vi "GetCameraData.vi"(7 "LabVIEW Web Service Request":refnum<class "Web Request.lvclass">) -> ()   [LabVIEW 2017]
uses:
  <vilib>/wsapi/Web Request.lvclass
  DataAccessors/action.ctl
  DataAccessors/cameraData.ctl
  DataAccessors/VisionWebServiceData.lvlib
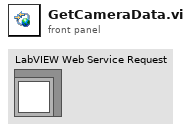
[diagram p1: front panel]
types:
  T1 = typedef "VisionWebServiceData.lvlib/action.ctl" = enum16{"Get", "Set"}
  T2 = typedef "VisionWebServiceData.lvlib/cameraData.ctl" = cluster{"Width":i32, "Height":i32, "Data":string}
  T3 = typedef "IrAcquisition.lvlib/camera.ctl" = cluster{"Name":string, "ChannelId":string, "CameraId":string, "SerialNumber":string, "Unit":string, "IMAQSession":T4, "InterfaceName":string, "RawImage":T5, "ScaledImage":T5, "TestPanelImage":T5, "Map":T6, "InDeviceModel":bool}
  T4 = typedef "IMAQdx.ctl" = refnum<k21>
  T5 = typedef "IMAQ Image.ctl" = refnum<image>
  T6 = typedef "PointValueMap.lvlib/PointMap.ctl" = refnum<data-value>
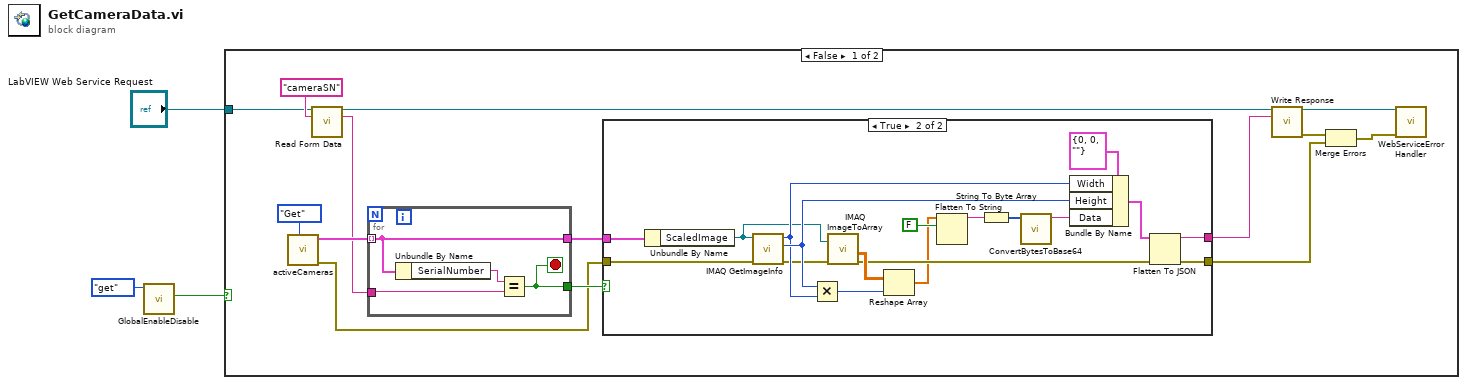
[diagram p0: block diagram]
diagram:
  n1 = call "GlobalEnableDisable.vi"("action"=enum16{"init", "set", "get"}."get") -> ("DisableDeviceWebService"=w1:bool)  [unwired: 10 in]
  n2 = case shown="False" w1 {
    tunnel: "LabVIEW Web Service Request" -> [w16 _]
    frame False {
      n3 = call "activeCameras.vi"("action"=action."Get") -> ("error out"=w7:errorcluster, "cameras"=w14:T3[])  [unwired: 9 in]
      n4 = call <vilib>:"Read Form Data.vi"("LabVIEW Web Service Request"=w16, "key"="cameraSN") -> ("LabVIEW Web Service Request out"=w13:refnum<class "Web Request.lvclass">, "value"=w8:string)  [unwired: 10 in, 2 out]
      n5 = for {
        tunnel: w14 -> [w38] mode=indexing
        tunnel: w8 -> [w39]
        tunnel: [w38] -> w10
        tunnel: [w37] -> w9
        stop <- w37 stop-if-true
        n6 = Unbundle By Name(w38) -> ("SerialNumber"=w40:string)
        n7 = Equal?(x=w40, y=w39) -> (x = y?=w37:bool)
      }
      n8 = case shown="True" w9 {
        tunnel: w10 -> [_ w36]
        tunnel: w7 -> [w18 w35]
        tunnel: [w18 w25] -> w6
        tunnel: [_ w20] -> w4
        frame False {
        }
        frame True {
          n9 = Unbundle By Name(w36) -> ("ScaledImage"=w29:T5)
          n10 = call "IMAQ GetImageInfo"("error in (no error)"=w35, "Image"=w29) -> ("error out"=w27:errorcluster, "Y Resolution"=w31:i32, "X Resolution"=w30:i32)  [unwired: 2 in, 5 out]
          n11 = Multiply(x=w31, y=w30) -> (x*y=w33:i32)
          n12 = call "IMAQ ImageToArray"("error in (no error)"=w27, "Image"=w29) -> ("Image Pixels (Float)"=w32:sgl[][], "error out"=w26:errorcluster)  [unwired: 2 in, 3 out]
          n13 = Reshape Array(w32, w33) -> (w21:sgl[])
          n14 = Flatten To String(anything=w21, prepend array or string size? (T)=FALSE) -> (data string=w22:string)  [unwired: 2 in, 2 out]
          n15 = String To Byte Array(string=w22) -> (unsigned byte array=w24:u8[])
          n16 = call <vilib>:"ConvertBytesToBase64.vi"("U8 array"=w24) -> ("base64 encoded"=w19:string)  [unwired: 10 in]
          n17 = Bundle By Name(cluster=T2 {"Width"=0, "Height"=0, "Data"=""} ("CameraData"), "Width"=w30, "Height"=w31, "Data"=w19) -> (w28:T2)
          n18 = Flatten To JSON(anything=w28, error in (no error)=w26) -> (JSON string=w20:string, 11:w25:errorcluster)  [unwired: 1 in]
        }
      }
      n19 = call <vilib>:"Write Response.vi"("LabVIEW Web Service Request"=w13, "response string"=w4) -> ("LabVIEW Web Service Request out"=w12:refnum<class "Web Request.lvclass">, "error out"=w5:errorcluster)  [unwired: 12 in]
      n20 = Merge Errors(w5, w6) -> (w11:errorcluster)
      n21 = call "WebServiceErrorHandler.vi"("LabVIEW Web Service Request"=w12, "error in (no error)"=w11) -> ()  [unwired: 12 in, 2 out]
    }
    frame True {
    }
  }
